vi "Initialize.vi"(8 "error in":errorcluster) -> (0 "error out":errorcluster, 3 "ChanMngOOB_Tx out":refnum<class "ChnMngOOB_Tx.lvclass">)   [LabVIEW 2021, in "ChnMngOOB_Tx.lvclass"]
uses:
  ChnMngOOB_Tx.lvclass
  C:/Program Files/National Instruments/LabVIEW 2021/vi.lib/CIF Foundation/CIF Out of Band Commands/CIFOutOfBand.lvclass
  Typedef/Template Payload.ctl
  typedef/Channel List for OOB.ctl
  <vilib>/CIF Foundation/CIF Channels Core/CIFChannels/Typedef/Direction.ctl
  Typedef/FIFO Publisher Return.ctl
  <vilib>/CIF Foundation/CIF Out of Band Commands/CIFOutOfBand.lvclass/CIFOutOfBand.ctl
  <vilib>/CIF Foundation/CIF Out of Band Commands/CIFOutOfBand.lvclass
  <vilib>/CIF Foundation/CIF Channels Core/CIFChannels/CIFChannels.lvclass
  CIFChannelMng.lvclass
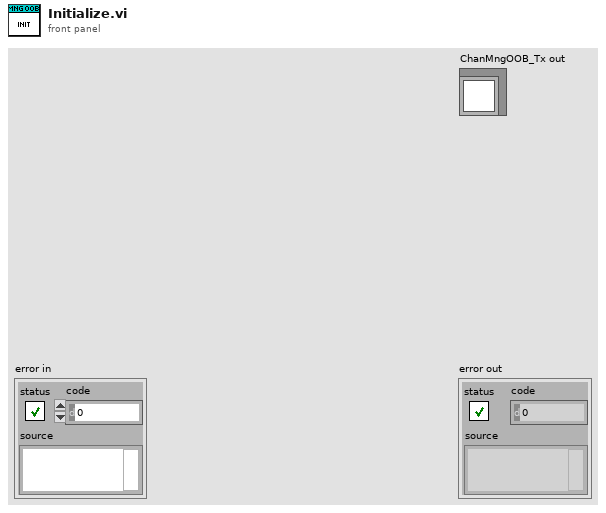
[diagram p1: front panel]
types:
  T1 = typedef "ChnMngOOB_Tx.lvclass/Template Payload.ctl" = cluster{"Channel List":T2[], "New FIFO Publisher":T4}
  T2 = typedef "CIFChannelMng.lvclass/Channel List for OOB.ctl" = cluster{"Name":string, "Direction":T3, "Type":string, "Connected?":bool, "Connected Name":string, "Custom Config Data":u8[], "Forced?":bool}
  T3 = typedef "CIFChannels.lvclass/Direction.ctl" = enum16{"Publisher", "Subscriber"}
  T4 = typedef "ChnMngOOB_Tx.lvclass/FIFO Publisher Return.ctl" = cluster{"FIFO Pub Name":string, "error":errorcluster, "Added":bool}
  T5 = typedef "ChnMngOOB_Tx.lvclass/OOB Core Commands.ctl" = enum8{"Channel List", "New FIFO Pub"}
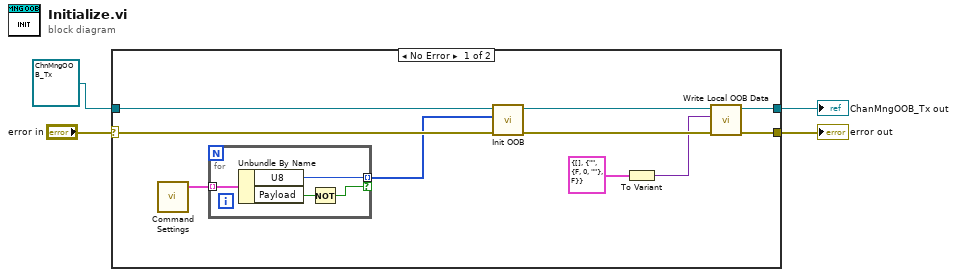
[diagram p0: block diagram]
diagram:
  n1 = case shown="No Error" "error in" {
    selector: "error in" -> [w14 w20]
    tunnel: [w8 w20] -> w3
    tunnel: [w7 w19] -> w2
    tunnel: refnum<class "ChnMngOOB_Tx.lvclass"> refnum ("CifLvTemplateOutOfBand in") -> [w13 w19]
    frame No Error {
      n2 = call "Command Settings.vi"() -> ("Command Stats"=w12:cluster{"Enum":T5, "U8":u8, "Payload":bool}[])  [unwired: 5 in]
      n3 = for {
        tunnel: w12 -> [w18] mode=indexing
        tunnel: [w17] -> w11 mode=indexing if=w15
        n4 = Unbundle By Name(w18) -> ("U8"=w17:u8, "Payload"=w16:bool)
        n5 = Not(x=w16) -> (.not. x?=w15:bool)
      }
      n6 = call <vilib>:"Init OOB.vi"("error in (no error)"=w14, "Cases to Skip Payload"=w11, "OOB in"=w13) -> ("error out"=w9:errorcluster, "OOB out"=w10:refnum<class "ChnMngOOB_Tx.lvclass">)  [unwired: 7 in]
      n7 = To Variant(anything=T1 {"Channel List"=[], "New FIFO Publisher"={"FIFO Pub Name"="", "error"={"status"=FALSE, "code"=0, "source"=""}, "Added"=FALSE}} ("Template Payload")) -> (Variant=w6:variant)
      n8 = call <vilib>:"Write Local OOB Data.vi"("error in"=w9, "Local OOB Data"=w6, "OOB in"=w10) -> ("error out"=w8:errorcluster, "OOB out"=w7:refnum<class "ChnMngOOB_Tx.lvclass">)  [unwired: 7 in]
    }
    frame Error {
    }
  }
  "error out" <- w3
  "ChanMngOOB_Tx out" <- w2
